vi "TurnOffDIO.vi"(8 "error in (no error)":errorcluster, 11 "DIOs to turn off":tag[](array[tag])) -> (0 "error out":errorcluster)   [LabVIEW 2014]
doc: "Sets specified DIO lines to false."
uses:
  <vilib>/DAQmx/create/channels.llb/DAQmx Create Channel (DO-Digital Output).vi
  <vilib>/DAQmx/write.llb/DAQmx Write (Digital Bool 1Line 1Point).vi
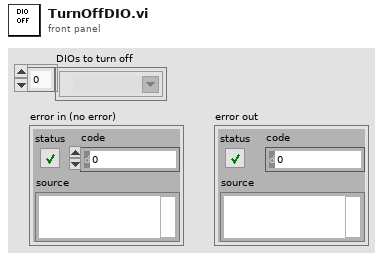
[diagram p1: front panel]
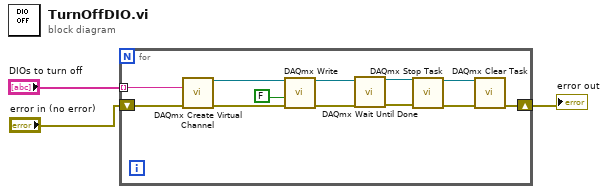
[diagram p0: block diagram]
diagram:
  n1 = for {
    tunnel: "DIOs to turn off" -> [w12] mode=indexing
    shift-right: [w4] -> w3
    shift-left: "error in (no error)" -> [w7]
    n2 = call-poly <vilib>:"DAQmx Create Virtual Channel.vi"("lines"=w12, "error in"=w7) -> ("task out"=w15:refnum<k21>, "error out"=w14:errorcluster)  [unwired: 12 in]
    n3 = call-poly <vilib>:"DAQmx Write.vi"("task/channels in"=w15, "data"=FALSE, "error in"=w14) -> ("task out"=w11:refnum<k21>, "error out"=w9:errorcluster)  [unwired: 1 in, 10 out]
    n4 = call <vilib>:"DAQmx Wait Until Done.vi"("task/channels in"=w11, "error in"=w9) -> ("task out"=w10:refnum<k21>, "error out"=w8:errorcluster)  [unwired: 12 in]
    n5 = call <vilib>:"DAQmx Stop Task.vi"("task/channels in"=w10, "error in"=w8) -> ("task out"=w5:refnum<k21>, "error out"=w6:errorcluster)  [unwired: 12 in]
    n6 = call <vilib>:"DAQmx Clear Task.vi"("task in"=w5, "error in"=w6) -> ("error out"=w4:errorcluster)  [unwired: 13 in]
  }
  "error out" <- w3
